vi "Multi-Channel Acquisition.vi"() -> ()   [LabVIEW 2018]
uses:
  Potentiostat Galvanostat Class/Controls/Channel.ctl
  Potentiostat Galvanostat Class/Controls/PEIS Parameters.ctl
  Potentiostat Galvanostat Class/Controls/GEIS Parameters.ctl
  Potentiostat Galvanostat Class/Controls/Technique List.ctl
  Potentiostat Galvanostat Class/Potentiostat Galvanostat.lvclass/Potentiostat Galvanostat.ctl
  Potentiostat Galvanostat Class/VIs/Set Channel.vi
  Potentiostat Galvanostat Class/VIs/Error Code Converter.vi
  Potentiostat Galvanostat Class/VIs/Insert Column into Table.vi
  Potentiostat Galvanostat Class/VIs/BL_GetErrorMsg.vi
  <vilib>/Utility/error.llb/Error Cluster From Error Code.vi
  Potentiostat Galvanostat Class/VIs/Get Enum Size.vi
  <vilib>/Utility/Data Type/Get Numeric Information.vi
  Potentiostat Galvanostat Class/Potentiostat Galvanostat.lvclass
panel:
  in  "stop 1":bool
  in  "stop 0":bool
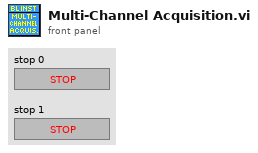
[diagram p1: front panel]
types:
  T1 = typedef "Potentiostat Galvanostat.lvclass/Technique List.ctl" = enum16{"None", "ocv", "cv", "biovscan", "ca", "cp", "iscan", "vscan", "lasv", "load", "pow", "peis", "geis", "seisp", "seisg", "dpv", "swv", "npv", "mpv", "dnpv", "dpa", "evt", "lp", "gc", "cpp", "pdp", "psp", "zra", "ircmp", "pzir", "gzir", "loop", "TO", "TI", "TOS", "vscanlimit", "iscanlimit", "mp", "casp", "casg", "calimit", "cplimit"}
  T2 = typedef "Potentiostat Galvanostat.lvclass/GEIS Parameters.ctl" = cluster{"Initial frequency (Hz)":sgl, "sweep linear/logarithmic":bool, "Number of frequencies":i32, "Final frequency (Hz)":sgl, "Sine amplitude (A)":sgl, "No. of repeat times":i32, "No. of period to wait\nbefore each frequency":sgl, "Non-stationary correction":bool, "I Range":u16, "Bandwidth":u16, "CE to ground Mode":u16, "Step duration (s)":sgl, "Record every dE (V)":sgl, "Record every dt (s)":sgl, "Initial current step (A)":sgl, "Current step vs initial one":bool}
  T3 = typedef "Potentiostat Galvanostat.lvclass/PEIS Parameters.ctl" = cluster{"Step duration (s)":sgl, "Record every dI (A)":sgl, "Record every dt (s)":sgl, "Initial voltage step (V)":sgl, "Voltage step vs initial one":bool, "Initial frequency (Hz)":sgl, "sweep linear/logarithmic":bool, "Number of frequencies":i32, "Final frequency (Hz)":sgl, "Sine amplitude (V)":sgl, "No. of repeat times":i32, "No. of period to wait\nbefore each frequency":sgl, "Non-stationary correction":bool, "I Range":u16, "Bandwidth":u16, "CE to ground Mode":u16}
  T4 = typedef "Potentiostat Galvanostat.lvclass/Channel.ctl" = u8
  T5 = typedef "Potentiostat Galvanostat.lvclass/Channel Data.ctl" = cluster{"Process Data":T6, "Data Information":T7, "Current Values":T9}
  T6 = typedef "Potentiostat Galvanostat.lvclass/Process Data.ctl" = cluster{"Process 0 Data":sgl[][], "Process 1 Data":sgl[][]}
  T7 = typedef "Potentiostat Galvanostat.lvclass/Data Information.ctl" = cluster{"Number of IRQ skipped":i32, "Buffer Row Size":i32, "Buffer Column Size":i32, "Technique Index":i32, "Technique ID":T8, "Process Index":i32, "Loop":i32, "Start Time (s)":sgl, "MuxPad":i32}
  T8 = typedef "Potentiostat Galvanostat.lvclass/Technique ID.ctl" = i32
  T9 = typedef "Potentiostat Galvanostat.lvclass/Current Values.ctl" = cluster{"State":T10, "Memory Filled (in Bytes)":i32, "Time Base (s)":sgl, "Ewe (V)":sgl, "Ewe Minimum Range (V)":sgl, "Ewe Maximum Range (V)":sgl, "Ece (V)":sgl, "Ece Minimum Range (V)":sgl, "Ece Maximum Range (V)":sgl, "E Overflow":i32, "I (A)":sgl, "I Range":T11, "I Overflow":i32, "Elapsed Time (s)":dbl, "Frequency (Hz)":sgl, "R Compensation (Ohm)":sgl, "E and/or I Saturation":sgl, "Hardware Option Error Code":T12, "Index of HW Option Error":i32}
  T10 = typedef "Potentiostat Galvanostat.lvclass/Channel State.ctl" = i32
  T11 = typedef "Potentiostat Galvanostat.lvclass/Current Range.ctl" = i32
  T12 = typedef "Potentiostat Galvanostat.lvclass/Error Codes.ctl" = i32
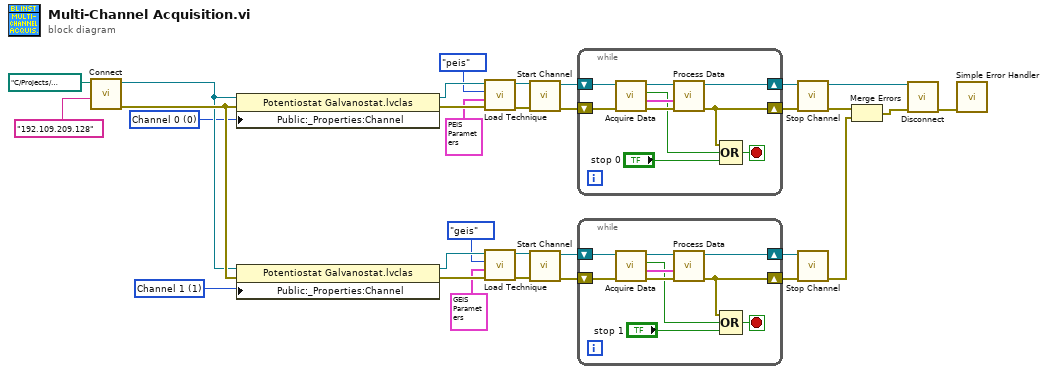
[diagram p0: block diagram]
diagram:
  w26 = T4 1 items=["Channel 0", "Channel 1", "Channel 2", "Channel 3", "Channel 4", "Channel 5", "Channel 6", "Channel 7", "Channel 8", "Channel 9", "Channel 10", "Channel 11", "Channel 12", "Channel 13", "Channel 14", "Channel 15"] ("Channel")
  w27 = T4 0 items=["Channel 0", "Channel 1", "Channel 2", "Channel 3", "Channel 4", "Channel 5", "Channel 6", "Channel 7", "Channel 8", "Channel 9", "Channel 10", "Channel 11", "Channel 12", "Channel 13", "Channel 14", "Channel 15"] ("Channel")
  n1 = call "Connect.vi"("IP Address/USB"="192.109.209.128", ".dll Path"=path "C:/Projects/LabVIEW/BioLogic Potentiostat Galvanostat Driver/src/support/libs/EC-Lab Development Package/EClib.dll" ("DLL Path in")) -> ("error out"=w31:errorcluster, "Potentiostat Galvanostat out"=w28:refnum<class "Potentiostat Galvanostat.lvclass">)  [unwired: 8 in]
  n2 = property class="Potentiostat Galvanostat.lvclas"(reference=w28, error in=w31, "Public:_Properties:Channel"=w27) -> (reference out=w22:refnum<class "Potentiostat Galvanostat.lvclass">, error out=w23:errorcluster)
  n3 = property class="Potentiostat Galvanostat.lvclas"(reference=w28, error in=w31, "Public:_Properties:Channel"=w26) -> (reference out=w8:refnum<class "Potentiostat Galvanostat.lvclass">, error out=w9:errorcluster)
  n4 = call "Load Technique.vi"("error in (no error)"=w23, "Technique Parameters in"=T3 {"Step duration (s)"=1.0, "Record every dI (A)"=0.1, "Record every dt (s)"=0.1, "Initial voltage step (V)"=0.0, "Voltage step vs initial one"=TRUE, "Initial frequency (Hz)"=100000.0, "sweep linear/logarithmic"=FALSE, "Number of frequencies"=51, "Final frequency (Hz)"=1.0, "Sine amplitude (V)"=0.01, "No. of repeat times"=1, "No. of period to wait\nbefore each frequency"=2.0, "Non-stationary correction"=TRUE, "I Range"=12, "Bandwidth"=5, "CE to ground Mode"=0} ("PEIS Parameters"), "Technique in"=Technique_List."peis", "Potentiostat Galvanostat in"=w22) -> ("error out"=w25:errorcluster, "Potentiostat Galvanostat out"=w24:refnum<class "Potentiostat Galvanostat.lvclass">)  [unwired: 6 in]
  n5 = call "Load Technique.vi"("error in (no error)"=w9, "Technique Parameters in"=T2 {"Initial frequency (Hz)"=100000.0, "sweep linear/logarithmic"=FALSE, "Number of frequencies"=51, "Final frequency (Hz)"=1.0, "Sine amplitude (A)"=0.001, "No. of repeat times"=1, "No. of period to wait\nbefore each frequency"=2.0, "Non-stationary correction"=TRUE, "I Range"=7, "Bandwidth"=5, "CE to ground Mode"=0, "Step duration (s)"=1.0, "Record every dE (V)"=0.1, "Record every dt (s)"=0.1, "Initial current step (A)"=0.0, "Current step vs initial one"=TRUE} ("GEIS Parameters"), "Technique in"=Technique_List."geis", "Potentiostat Galvanostat in"=w8) -> ("error out"=w15:errorcluster, "Potentiostat Galvanostat out"=w14:refnum<class "Potentiostat Galvanostat.lvclass">)  [unwired: 6 in]
  n6 = call "Start Channel.vi"("error in (no error)"=w25, "Potentiostat Galvanostat in"=w24) -> ("error out"=w20:errorcluster, "Potentiostat Galvanostat out"=w21:refnum<class "Potentiostat Galvanostat.lvclass">)  [unwired: 8 in]
  n7 = call "Start Channel.vi"("error in (no error)"=w15, "Potentiostat Galvanostat in"=w14) -> ("error out"=w12:errorcluster, "Potentiostat Galvanostat out"=w13:refnum<class "Potentiostat Galvanostat.lvclass">)  [unwired: 8 in]
  n8 = while {
    shift-right: [w36] -> w19
    shift-left: w21 -> [w38]
    shift-right: [w34] -> w18
    shift-left: w20 -> [w37]
    stop <- w32 stop-if-true
    n9 = call "Acquire Data.vi"("error in (no error)"=w37, "Potentiostat Galvanostat in"=w38) -> ("error out"=w41:errorcluster, "Channel Data"=w39:T5, "Finished?"=w33:bool, "Potentiostat Galvanostat out"=w40:refnum<class "Potentiostat Galvanostat.lvclass">)  [unwired: 6 in]
    n10 = call "Process Data.vi"("error in (no error)"=w41, "Channel Data"=w39, "Potentiostat Galvanostat in"=w40) -> ("error out"=w34:errorcluster, "Potentiostat Galvanostat out"=w36:refnum<class "Potentiostat Galvanostat.lvclass">)  [unwired: 5 in, 2 out]
    n11 = Compound Arithmetic op=OR(w34, w33, "stop 0") -> (w32:bool)
  }
  n12 = while {
    shift-right: [w46] -> w11
    shift-left: w13 -> [w48]
    shift-right: [w44] -> w10
    shift-left: w12 -> [w47]
    stop <- w42 stop-if-true
    n13 = call "Acquire Data.vi"("error in (no error)"=w47, "Potentiostat Galvanostat in"=w48) -> ("error out"=w51:errorcluster, "Channel Data"=w49:T5, "Finished?"=w43:bool, "Potentiostat Galvanostat out"=w50:refnum<class "Potentiostat Galvanostat.lvclass">)  [unwired: 6 in]
    n14 = call "Process Data.vi"("error in (no error)"=w51, "Channel Data"=w49, "Potentiostat Galvanostat in"=w50) -> ("error out"=w44:errorcluster, "Potentiostat Galvanostat out"=w46:refnum<class "Potentiostat Galvanostat.lvclass">)  [unwired: 5 in, 2 out]
    n15 = Compound Arithmetic op=OR(w44, w43, "stop 1") -> (w42:bool)
  }
  n16 = call "Stop Channel.vi"("error in (no error)"=w18, "Potentiostat Galvanostat in"=w19) -> ("error out"=w4:errorcluster, "Potentiostat Galvanostat out"=w2:refnum<class "Potentiostat Galvanostat.lvclass">)  [unwired: 8 in]
  n17 = call "Stop Channel.vi"("error in (no error)"=w10, "Potentiostat Galvanostat in"=w11) -> ("error out"=w3:errorcluster)  [unwired: 8 in, 1 out]
  n18 = Merge Errors(w4, w3) -> (w1:errorcluster)
  n19 = call "Disconnect.vi"("error in (no error)"=w1, "Potentiostat Galvanostat in"=w2) -> ("error out"=w5:errorcluster)  [unwired: 9 in]
  n20 = call <vilib>:"Simple Error Handler.vi"("error in (no error)"=w5) -> ()  [unwired: 4 in, 5 out]
